vi "Main.vi"() -> ()   [LabVIEW 2013]
uses:
  <vilib>/Analysis/NI_AALBase.lvlib
  <vilib>/Analysis/1siggen.llb/Ramp Pattern by Samples.vi
  <vilib>/DAQmx/create/channels.llb/DAQmx Create Channel (AO-Voltage-Basic).vi
  <vilib>/DAQmx/write.llb/DAQmx Write (Analog 1D DBL NChan 1Samp).vi
panel:
  in  "Define as center":bool
  out "Voltage out":dbl[](array[numeric])
  in  "Relative Position":cluster{"X":i32, "Y":i32, "Z":i32}
  in  "Voltage Step":cluster{"X":dbl, "Y":dbl, "Z":dbl}
  in  "Center Voltage":cluster{"X":dbl, "Y":dbl, "Z":dbl}
  in  "2nd Dim":u32
  in  "3rd Dim":u32
  out "Intensity Graph":dbl[][](graph)
  out "XY Graph":T1(graph)
  out "Scanning":bool
  out "Estimated Time (ms)":dbl
  in  "dt (in tc)":u32
  in  "Dim3Scan":cluster{"Start":dbl, "Stop":dbl, "Steps":u32}
  in  "Dim3":u16(ring) items=["Z", "none"]
  in  "Dim2Scan":cluster{"Start":dbl, "Stop":dbl, "Steps":u32}
  in  "Dim2":u16(ring) items=["Y", "Z", "none"]
  in  "Dim1Scan":cluster{"Start":dbl, "Stop":dbl, "Steps":u32}
  in  "Dim1":u16(ring) items=["X", "Y", "Z"]
  in  "Start Scan":bool
  out "Error":errorcluster
  out "History Graph":cluster{dbl[], dbl[]}(graph)
  in  "N":u32
  out "Value":dbl
  in  "tc (ms)":u32
  in  "stop":bool
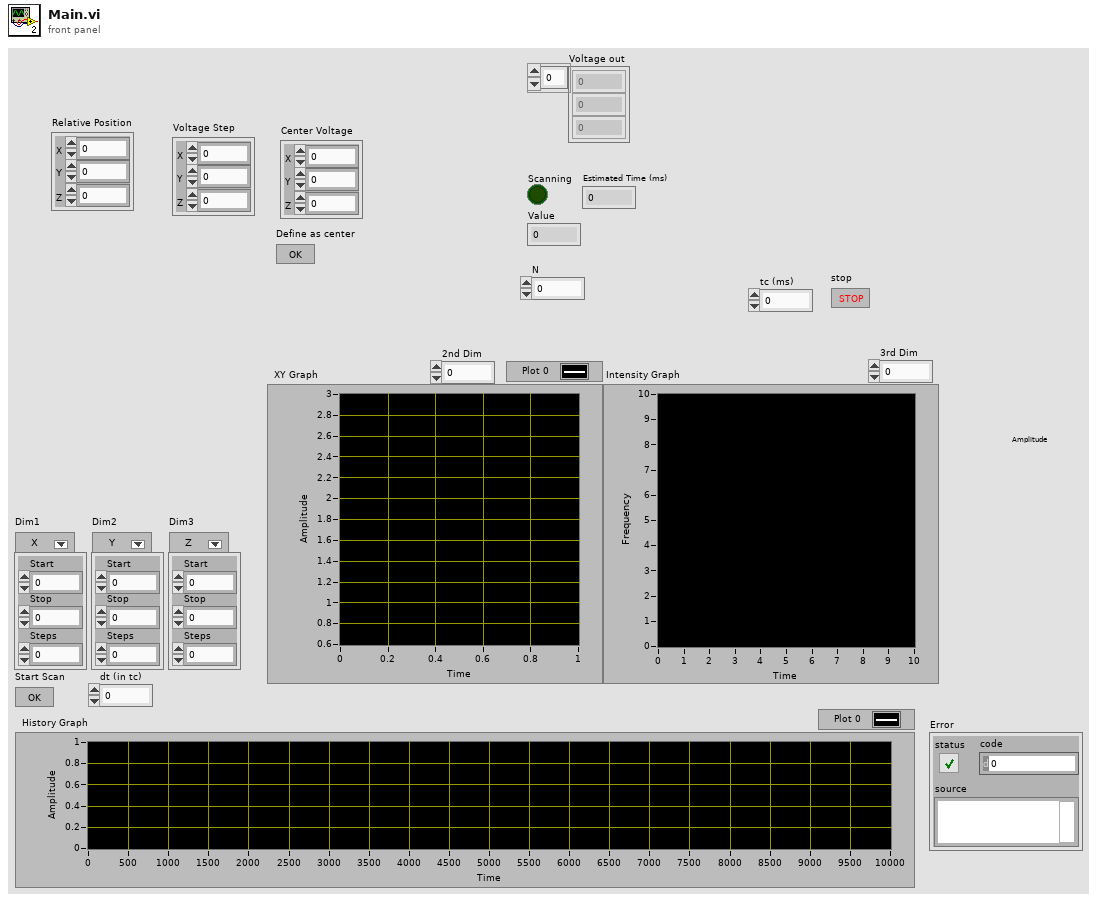
[diagram p1: front panel]
types:
  T1 = cluster{"Ramp Pattern":dbl[], "Ramp Pattern":dbl[]}
  T2 = enum16{"open", "replace", "create", "open or create", "replace or create", "replace or create with confirmation"}
  T3 = cluster{"Ramp Pattern":dbl[], "initialized array":dbl[]}
  T4 = cluster{"Voltage out[0]":dbl, "Voltage out[1]":dbl, "Voltage out[2]":dbl}
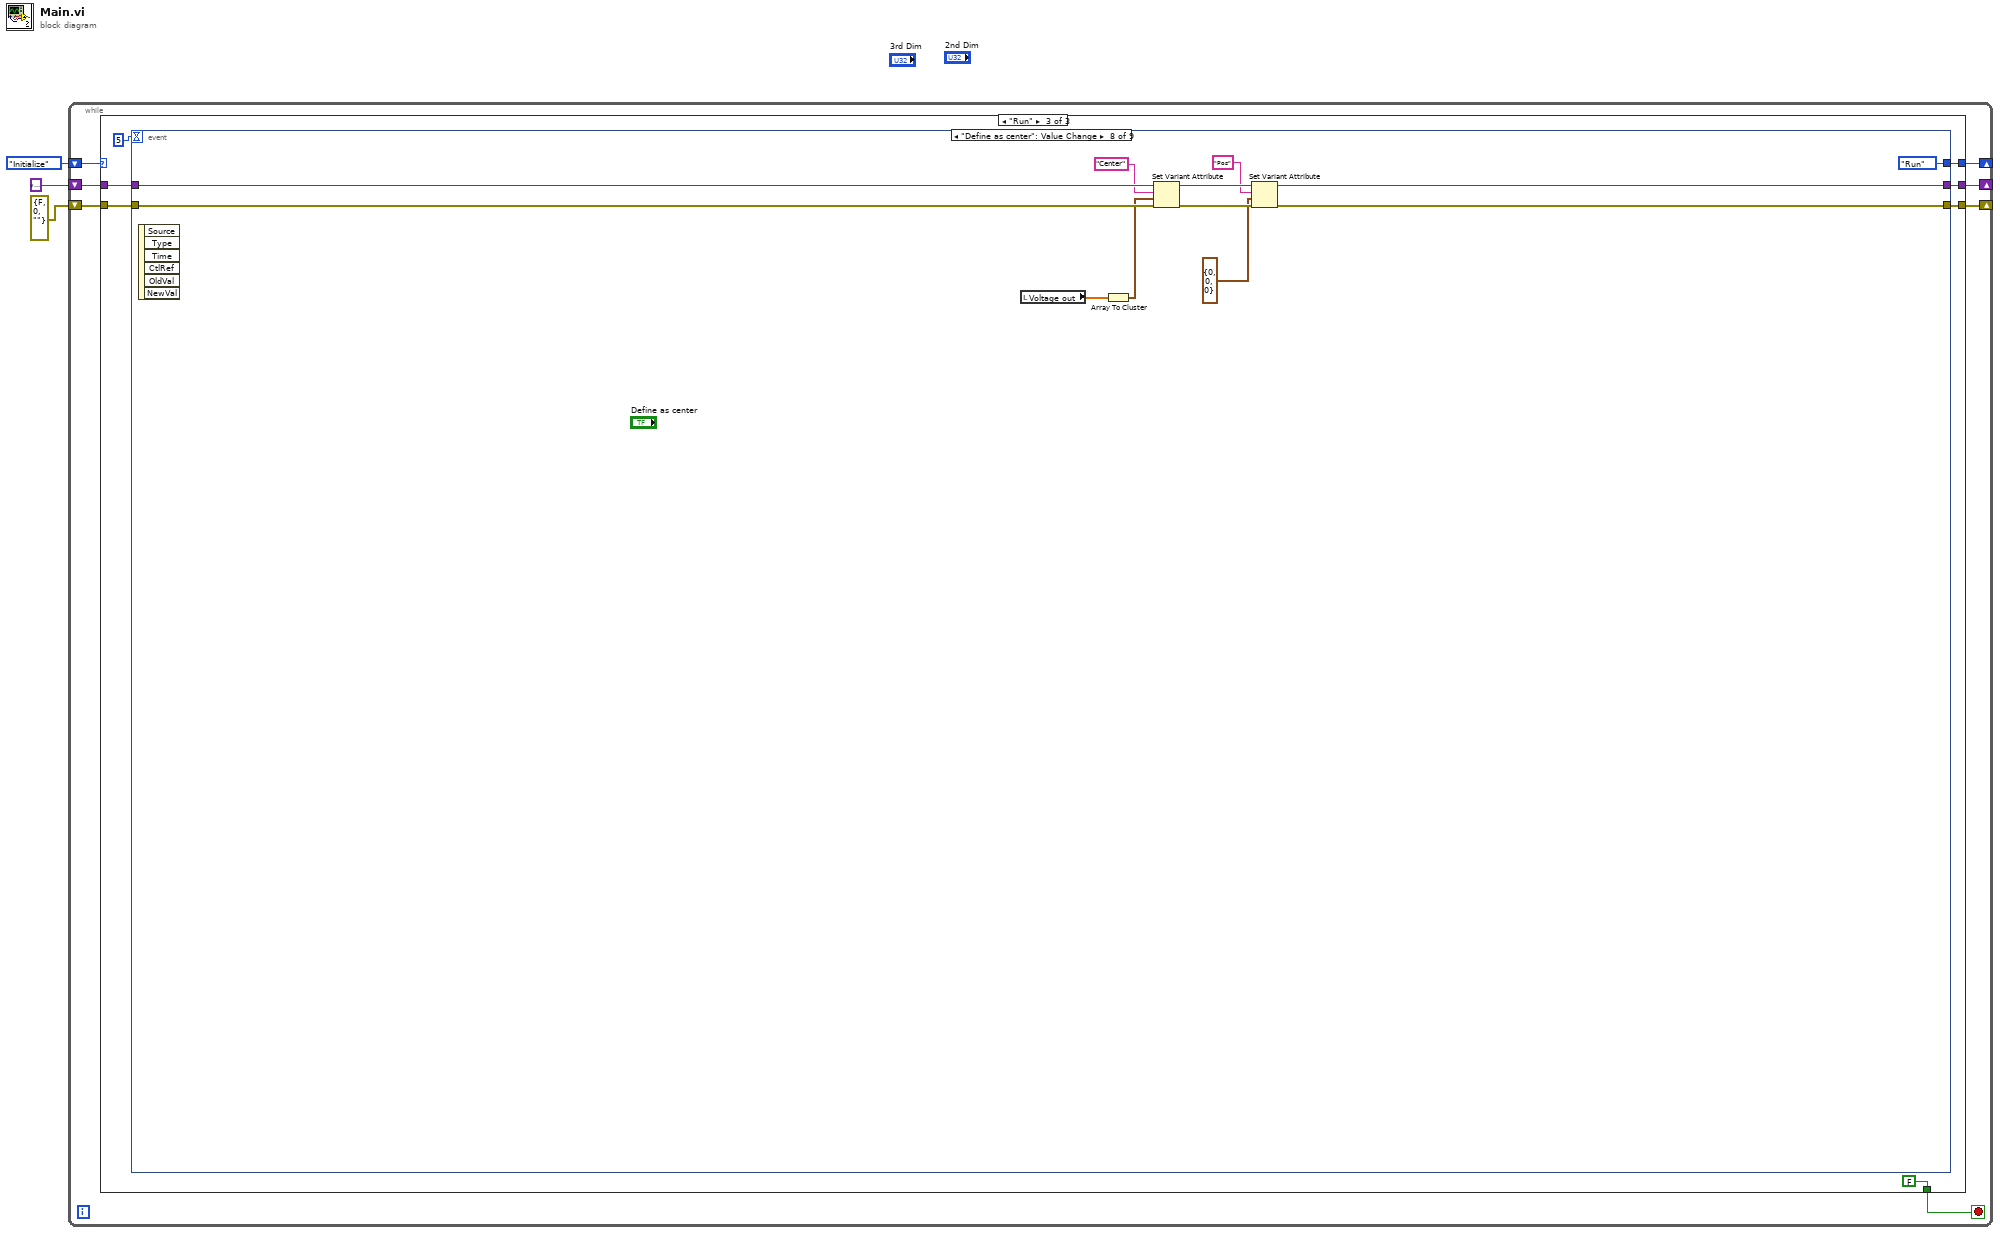
[diagram p0: block diagram]
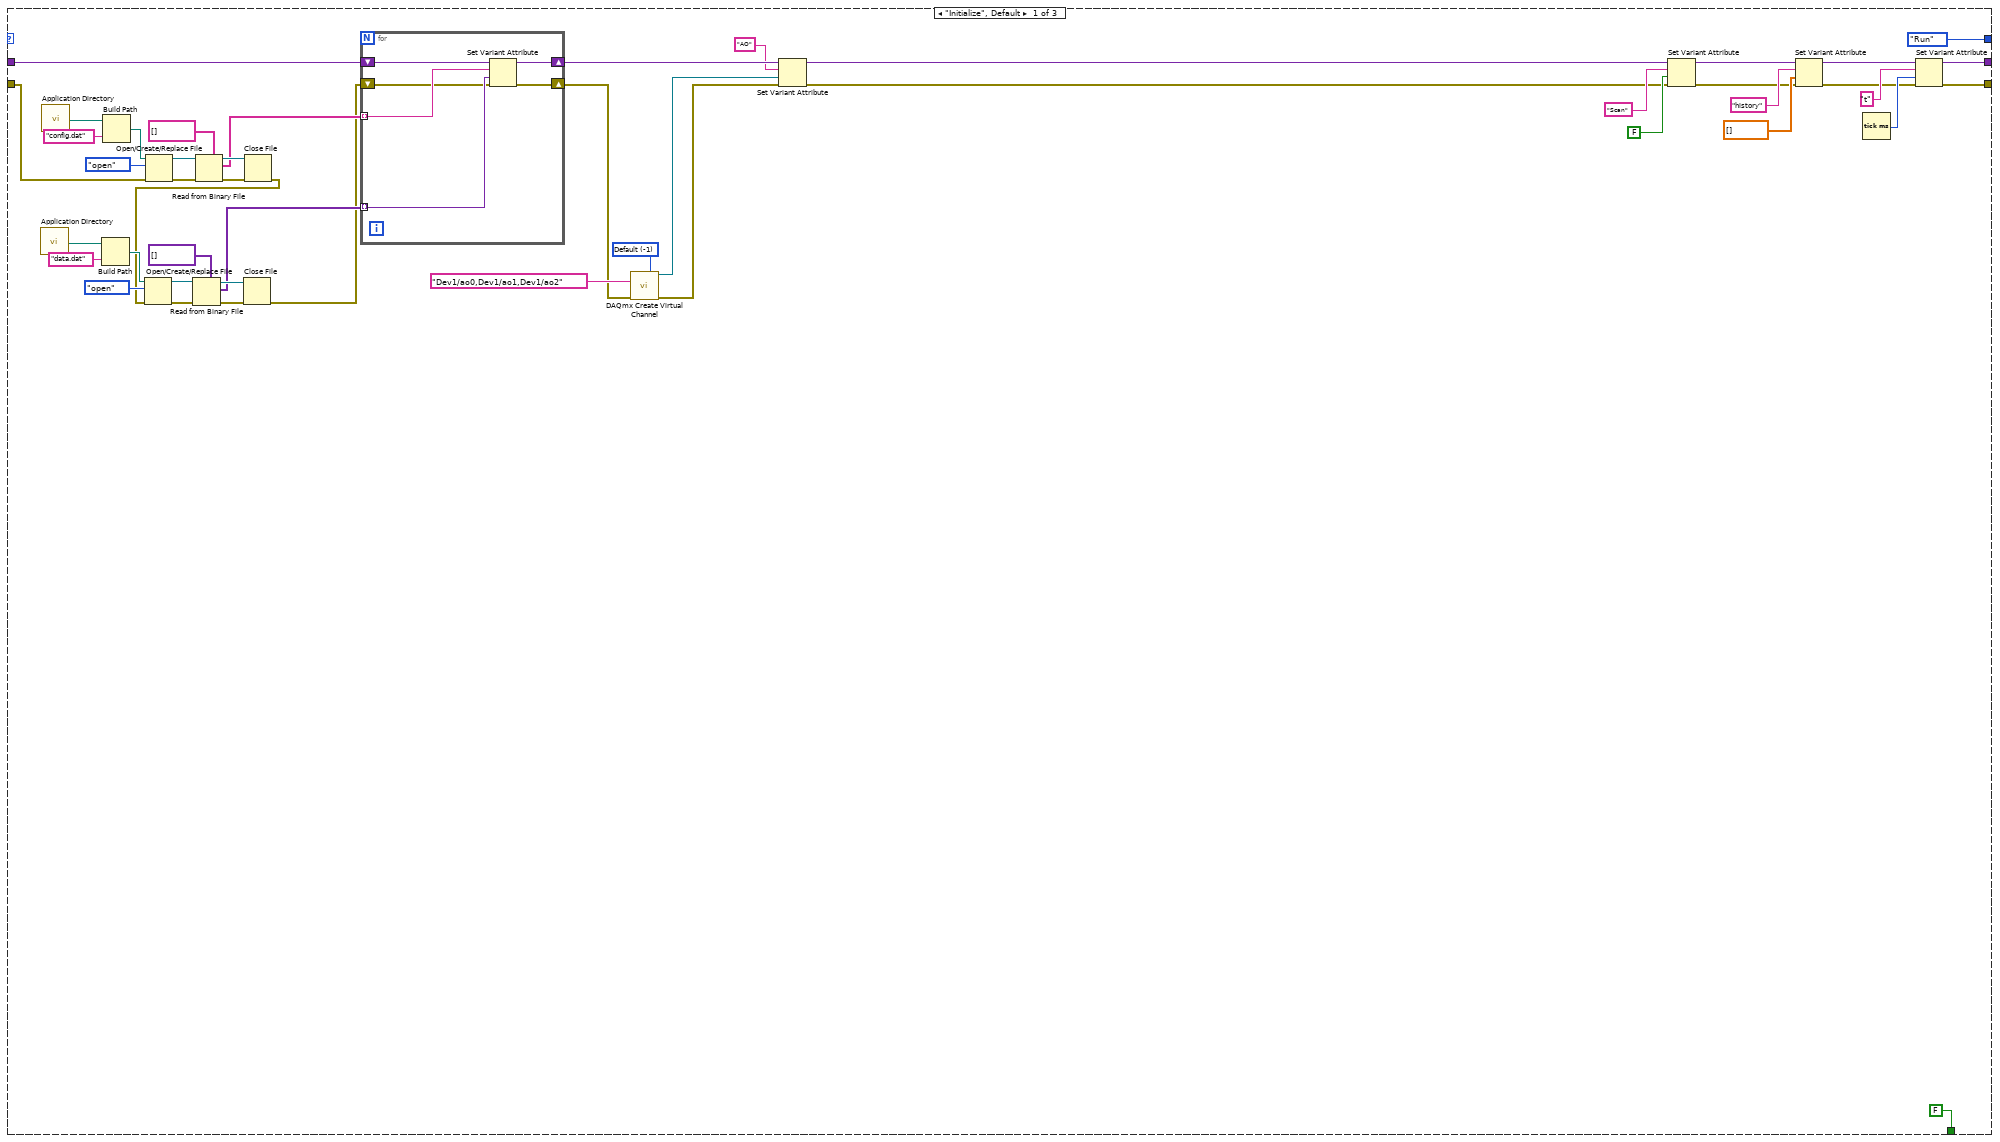
[diagram p2: hidden frame]
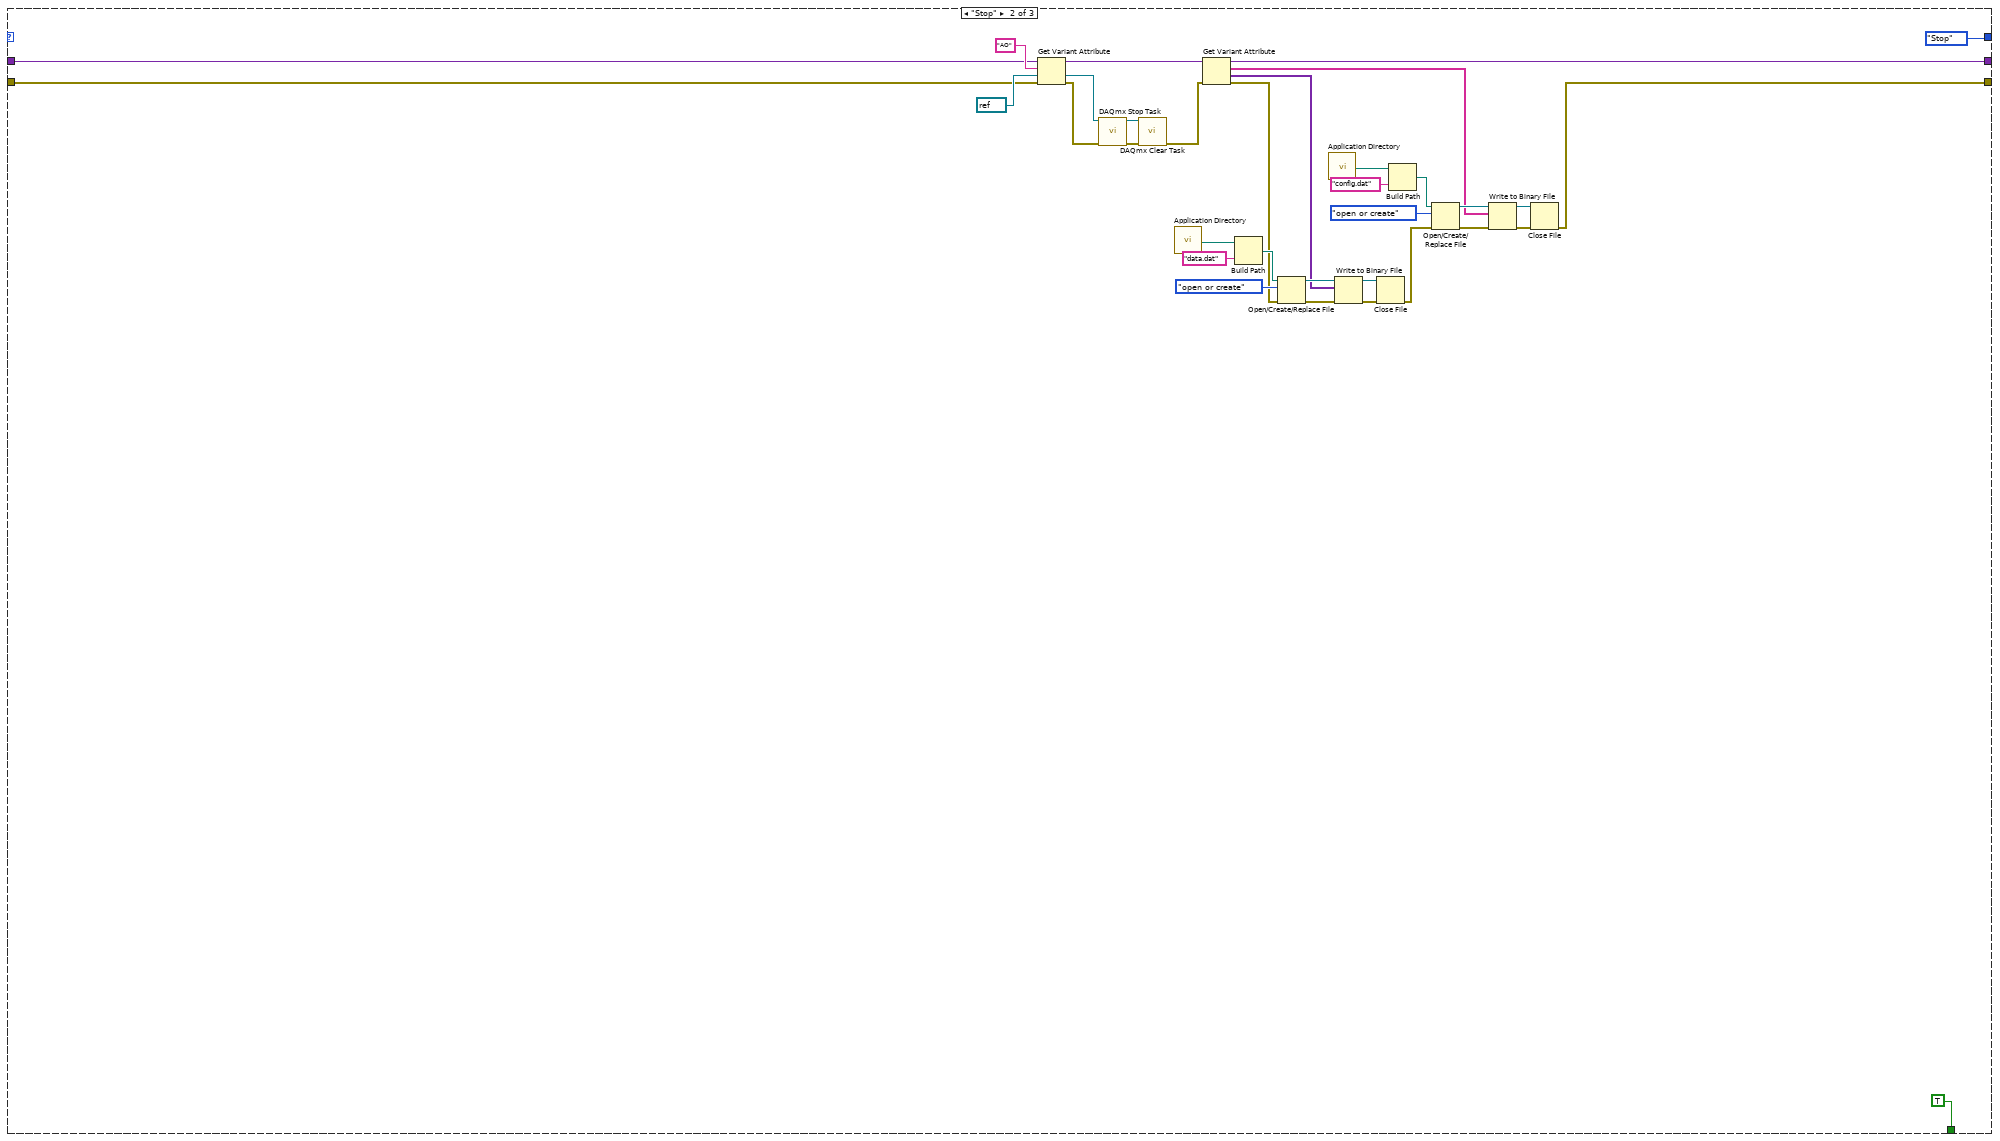
[diagram p3: hidden frame]
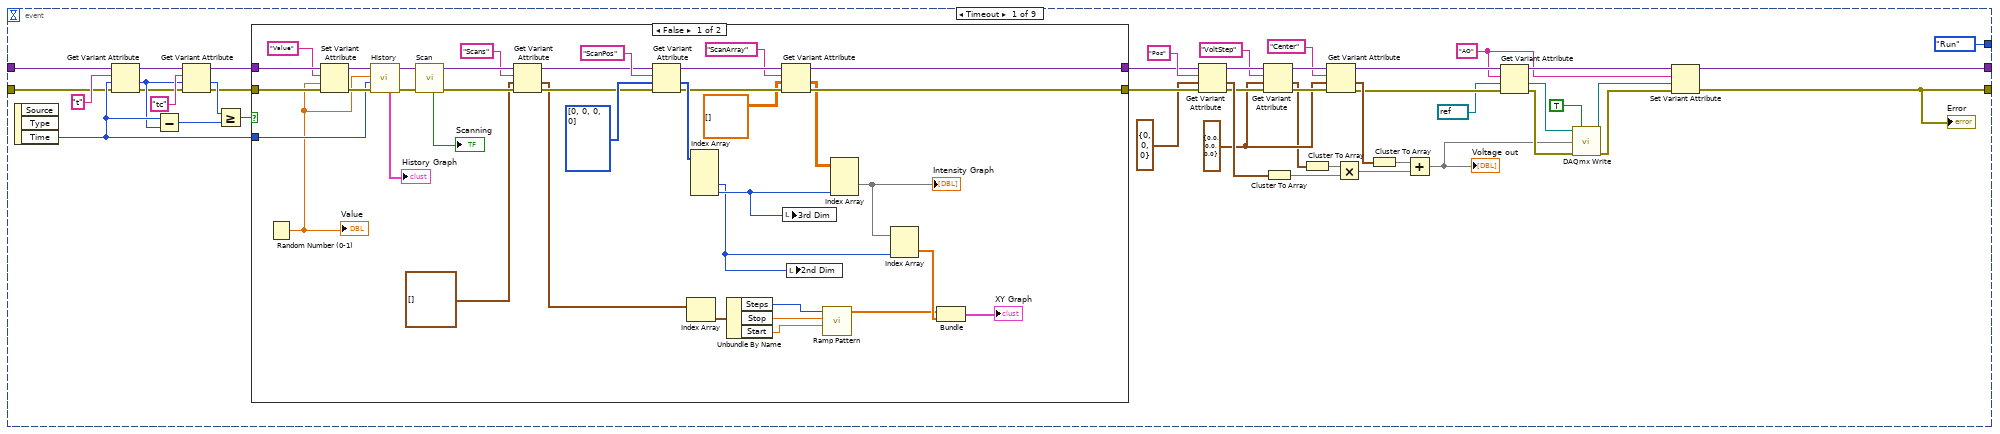
[diagram p4: hidden frame]
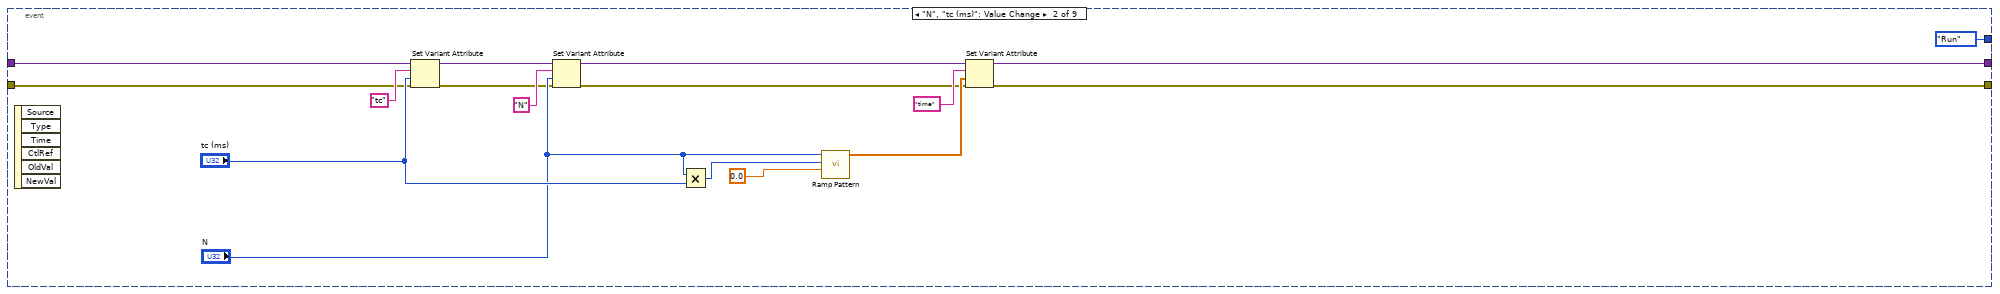
[diagram p6: hidden frame]
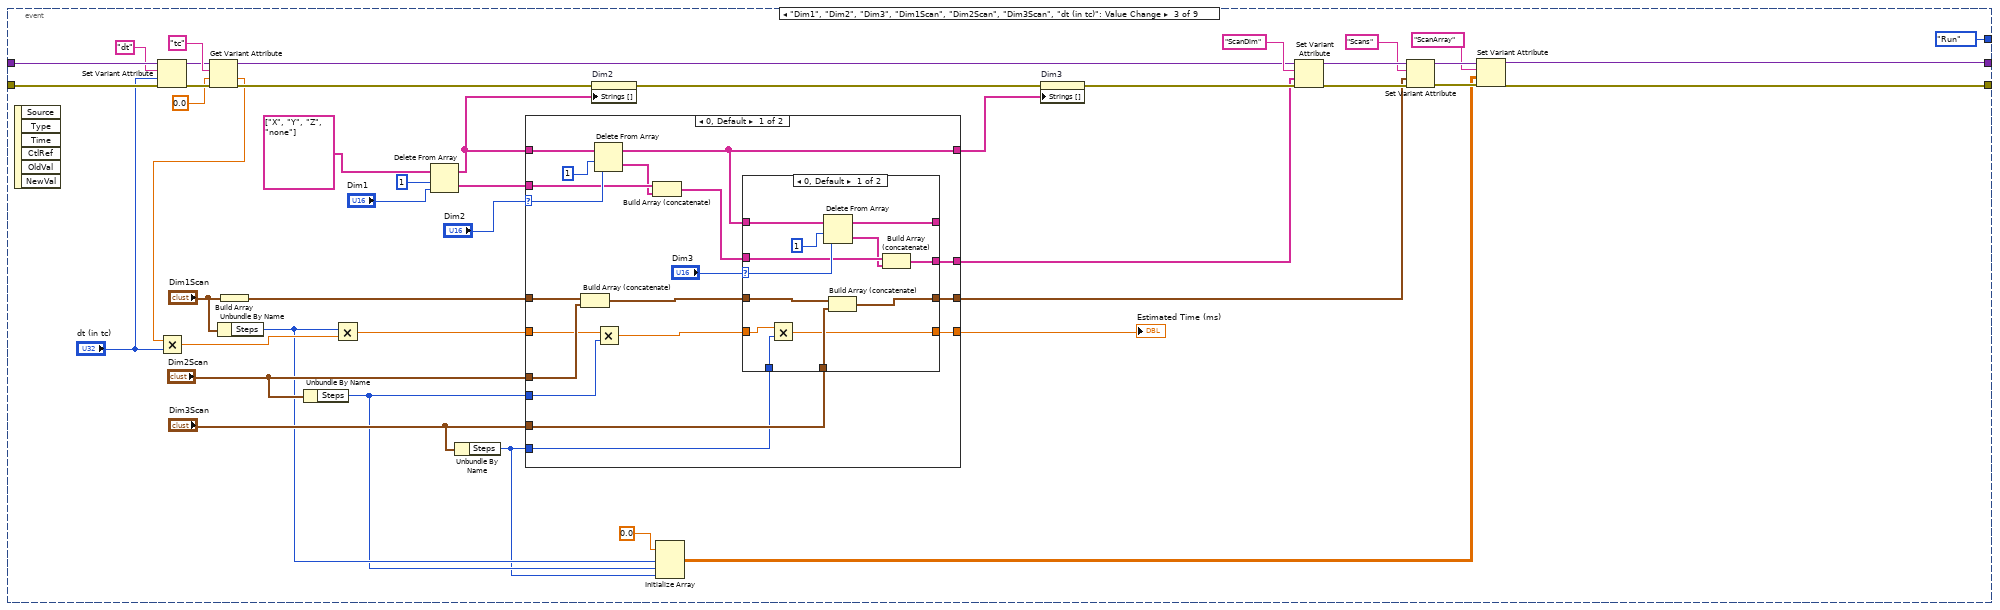
[diagram p7: hidden frame]
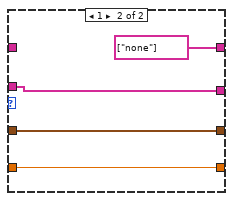
[diagram p8: hidden frame]
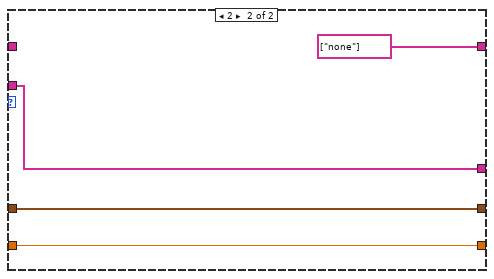
[diagram p9: hidden frame]
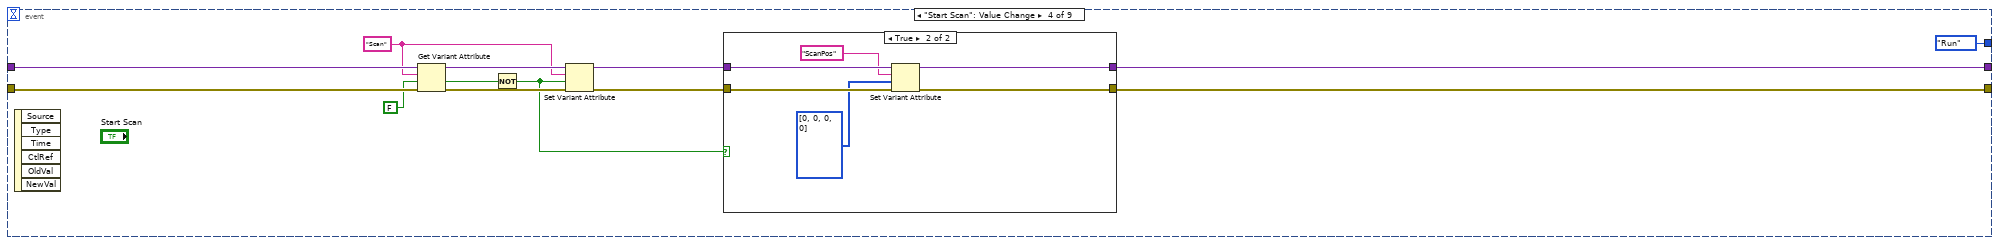
[diagram p10: hidden frame]
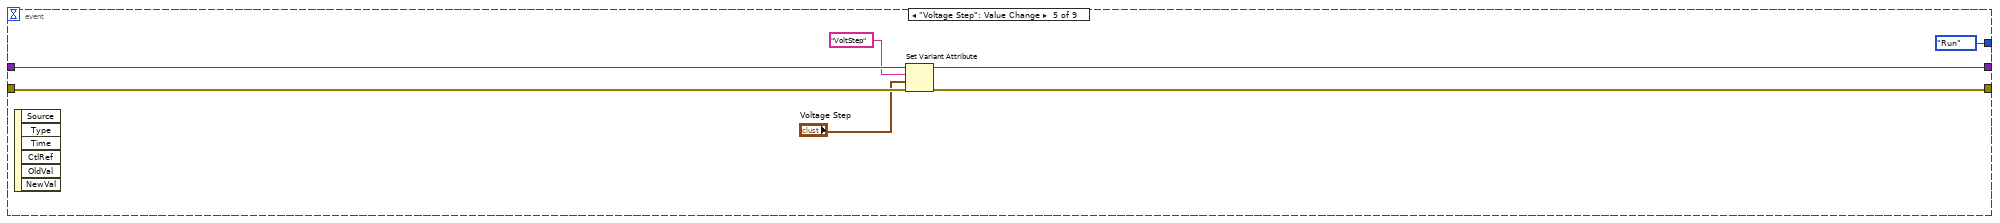
[diagram p12: hidden frame]
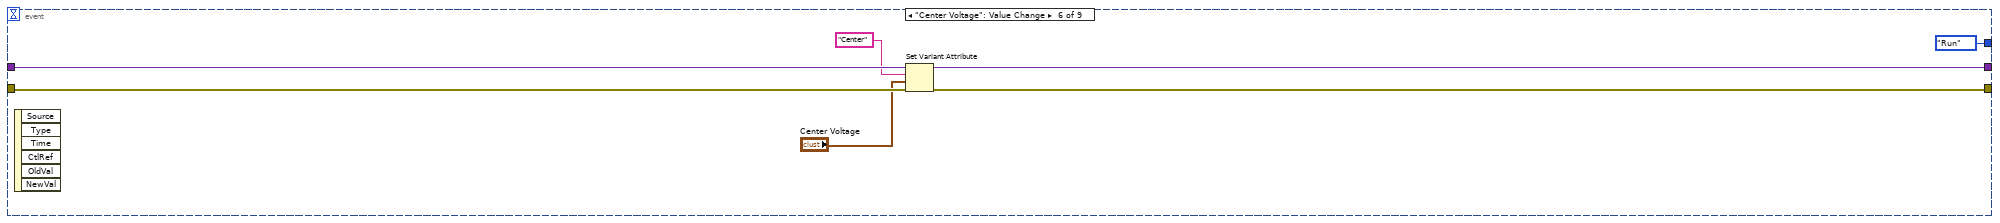
[diagram p13: hidden frame]
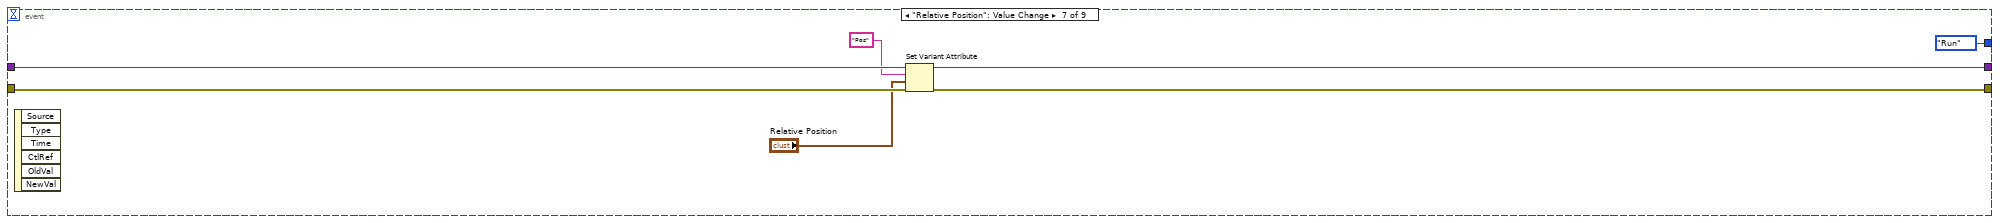
[diagram p14: hidden frame]
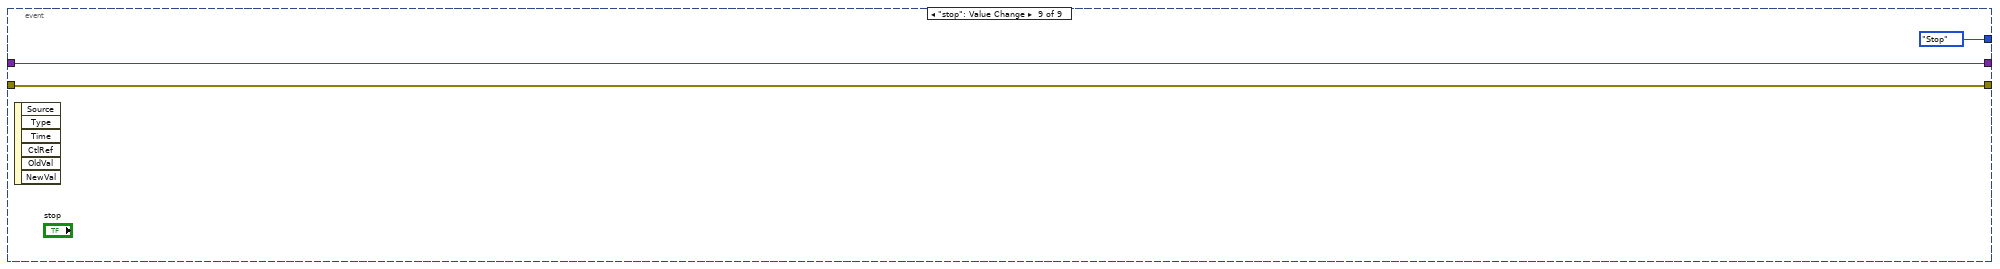
[diagram p15: hidden frame]
diagram:
  n1 = while {
    shift-right: [w9] -> _
    shift-left: enum16{"Initialize", "Run", "Stop"}."Initialize" -> [w10]
    shift-right: [w5] -> _
    shift-left: variant ("variant") -> [w7]
    shift-right: [w4] -> _
    shift-left: errorcluster {"status"=FALSE, "code"=0, "source"=""} ("error constant") -> [w6]
    stop <- w8 stop-if-true
    n2 = case shown="\"Run\"" w10 {
      tunnel: [enum16{"Initialize", "Run", "Stop"}."Run" enum16{"Initialize", "Run", "Stop"}."Stop" w104] -> w9
      tunnel: [FALSE TRUE FALSE] -> w8
      tunnel: w7 -> [w25 w70 w101]
      tunnel: w6 -> [w24 w69 w100]
      tunnel: [w27 w74 w99] -> w5
      tunnel: [w26 w75 w98] -> w4
      frame "Initialize", Default {
        w11 = -1 items=["Default"=-1, "RSE"=10083, "Differential"=10106, "Pseudodifferential"=12529] ("output terminal configuration")
        n3 = call <vilib>:"Application Directory.vi"() -> ("Application Directory"=w43:path)
        n4 = call <vilib>:"Application Directory.vi"() -> ("Application Directory"=w50:path)
        n5 = Build Path(base path=w43, name or relative path="data.dat") -> (appended path=w45:path)
        n6 = Build Path(base path=w50, name or relative path="config.dat") -> (appended path=w48:path)
        n7 = Open/Create/Replace File(file path (use dialog)=w48, error in=w24, operation (0:open)=T2."open") -> (refnum out=w40:refnum<file>, error out=w39:errorcluster)  [unwired: 3 in, 1 out]
        n8 = Read from Binary File(5:string[] [] ("names"), 8:w39, 11:w40) -> (0:w42:errorcluster, 2:w32:string[], 3:w41:refnum<file>)  [unwired: 3 in, 1 out]
        n9 = Close File(refnum=w41, error in=w42) -> (error out=w29:errorcluster)  [unwired: 1 out]
        n10 = Open/Create/Replace File(file path (use dialog)=w45, error in=w29, operation (0:open)=T2."open") -> (refnum out=w37:refnum<file>, error out=w38:errorcluster)  [unwired: 3 in, 1 out]
        n11 = Read from Binary File(5:variant[] [] ("values"), 8:w38, 11:w37) -> (0:w35:errorcluster, 2:w31:variant[], 3:w36:refnum<file>)  [unwired: 3 in, 1 out]
        n12 = Close File(refnum=w36, error in=w35) -> (error out=w28:errorcluster)  [unwired: 1 out]
        n13 = for {
          tunnel: w32 -> [w61] mode=indexing
          tunnel: w31 -> [w60] mode=indexing
          shift-right: [w62] -> w17
          shift-left: w25 -> [w63]
          shift-right: [w59] -> w18
          shift-left: w28 -> [w58]
          n14 = Set Variant Attribute(Variant=w63, name=w61, value=w60, error in=w58) -> (Variant out=w62:variant, error out=w59:errorcluster)  [unwired: 1 out]
        }
        n15 = call-poly <vilib>:"DAQmx Create Virtual Channel.vi"("output terminal configuration"=w11, "physical channels"=tag "Dev1/ao0,Dev1/ao1,Dev1/ao2", "error in"=w18) -> ("task out"=w15:refnum<k21>, "error out"=w16:errorcluster)  [unwired: 11 in]
        n16 = Set Variant Attribute(Variant=w17, name="AO", value=w15, error in=w16) -> (Variant out=w13:variant, error out=w12:errorcluster)  [unwired: 1 out]
        n17 = Set Variant Attribute(Variant=w13, name="Scan", value=FALSE, error in=w12) -> (Variant out=w23:variant, error out=w22:errorcluster)  [unwired: 1 out]
        n18 = Set Variant Attribute(Variant=w23, name="history", value=dbl[] [], error in=w22) -> (Variant out=w53:variant, error out=w30:errorcluster)  [unwired: 1 out]
        n19 = Tick Count (ms)() -> (millisecond timer value=w54:u32)
        n20 = Set Variant Attribute(Variant=w53, name="t", value=w54, error in=w30) -> (Variant out=w27:variant, error out=w26:errorcluster)  [unwired: 1 out]
      }
      frame "Stop" {
        n21 = Get Variant Attribute(Variant=w70, name="AO", default value (empty Variant)=refnum<k21> refnum ("task out"), error in=w69) -> (duplicate Variant=w71:variant, value=w64:refnum<k21>, error out=w66:errorcluster)  [unwired: 1 out]
        n22 = call <vilib>:"DAQmx Stop Task.vi"("task/channels in"=w64, "error in"=w66) -> ("task out"=w68:refnum<k21>, "error out"=w67:errorcluster)  [unwired: 12 in]
        n23 = call <vilib>:"DAQmx Clear Task.vi"("task in"=w68, "error in"=w67) -> ("error out"=w65:errorcluster)  [unwired: 13 in]
        n24 = call <vilib>:"Application Directory.vi"() -> ("Application Directory"=w88:path)
        n25 = Get Variant Attribute(Variant=w71, error in=w65) -> (duplicate Variant=w74:variant, names=w78:string[], values=w87:variant[], error out=w77:errorcluster)  [unwired: 2 in]
        n26 = Build Path(base path=w88, name or relative path="data.dat") -> (appended path=w94:path)
        n27 = Open/Create/Replace File(file path (use dialog)=w94, error in=w77, operation (0:open)=T2."open or create") -> (refnum out=w93:refnum<file>, error out=w90:errorcluster)  [unwired: 3 in, 1 out]
        n28 = call <vilib>:"Application Directory.vi"() -> ("Application Directory"=w86:path)
        n29 = Write to Binary File(file (use dialog)=w93, data=w87, error in=w90) -> (refnum out=w91:refnum<file>, error out=w89:errorcluster)  [unwired: 3 in, 1 out]
        n30 = Close File(refnum=w91, error in=w89) -> (error out=w76:errorcluster)  [unwired: 1 out]
        n31 = Build Path(base path=w86, name or relative path="config.dat") -> (appended path=w80:path)
        n32 = Open/Create/Replace File(file path (use dialog)=w80, error in=w76, operation (0:open)=T2."open or create") -> (refnum out=w81:refnum<file>, error out=w84:errorcluster)  [unwired: 3 in, 1 out]
        n33 = Write to Binary File(file (use dialog)=w81, data=w78, error in=w84) -> (refnum out=w83:refnum<file>, error out=w85:errorcluster)  [unwired: 3 in, 1 out]
        n34 = Close File(refnum=w83, error in=w85) -> (error out=w75:errorcluster)  [unwired: 1 out]
      }
      frame "Run" {
        n35 = event shown="[7] \"Define as center\": Value Change" {
          selector: _ -> [_ _ _ _ _ _ _ _ _]
          dyn-events: _ -> [_ _ _ _ _ _ _ _ _]
          timeout: 5 -> [_ _ _ _ _ _ _ _ _]
          tunnel: [enum16{"Initialize", "Run", "Stop"}."Run" enum16{"Initialize", "Run", "Stop"}."Run" enum16{"Initialize", "Run", "Stop"}."Run" enum16{"Initialize", "Run", "Stop"}."Run" enum16{"Initialize", "Run", "Stop"}."Run" enum16{"Initialize", "Run", "Stop"}."Run" enum16{"Initialize", "Run", "Stop"}."Run" enum16{"Initialize", "Run", "Stop"}."Run" enum16{"Initialize", "Run", "Stop"}."Stop"] -> w104
          tunnel: w101 -> [w139 w193 w235 w302 w317 w324 w331 w343 w346]
          tunnel: w100 -> [w138 w192 w234 w301 w316 w323 w330 w341 w345]
          tunnel: [w106 w191 w210 w292 w315 w322 w329 w340 w346] -> w99
          tunnel: [w105 w190 w209 w291 w314 w321 w328 w339 w345] -> w98
          event Timeout {
            w107 = "AO" ("name")
            w124 = cluster{"X":dbl, "Y":dbl, "Z":dbl} {"X"=0.0, "Y"=0.0, "Z"=0.0} ("Relative Position")
            n36 = event-data() -> ("Time"=w145:u32)  [unwired: 1 in, 2 out]
            n37 = Get Variant Attribute(Variant=w139, name="t", default value (empty Variant)=w145, error in=w138) -> (duplicate Variant=w144:variant, value=w142:u32, error out=w140:errorcluster)  [unwired: 1 out]
            n38 = Subtract(x=w145, y=w142) -> (x-y=w147:u32)
            n39 = Get Variant Attribute(Variant=w144, name="tc", default value (empty Variant)=w142, error in=w140) -> (duplicate Variant=w137:variant, value=w141:u32, error out=w136:errorcluster)  [unwired: 1 out]
            n40 = Greater Or Equal?(x=w141, y=w147) -> (x >= y?=w146:bool)
            n41 = case shown="False" w146 {
              tunnel: w145 -> [w181 _]
              tunnel: w137 -> [w187 w189]
              tunnel: w136 -> [w186 w188]
              tunnel: [w171 w189] -> w134
              tunnel: [w170 w188] -> w133
              frame False {
                n42 = Random Number (0-1)() -> (number: 0 to 1=w180:dbl)
                "Value" <- w180
                n43 = Set Variant Attribute(Variant=w187, name="Value", value=w180, error in=w186) -> (Variant out=w183:variant, error out=w184:errorcluster)  [unwired: 1 out]
                n44 = call "History.vi"("error in"=w184, "time"=w181, "Value"=w180, "variant in"=w183) -> ("error out"=w178:errorcluster, "variant out"=w179:variant, "history graph"=→"History Graph":cluster{dbl[], dbl[]})  [unwired: 5 in]
                n45 = call "Scan.vi"("error in"=w178, "variant in"=w179) -> ("error out"=w164:errorcluster, "variant out"=w165:variant, "Scanning"=→"Scanning":bool)  [unwired: 7 in]
                n46 = Get Variant Attribute(Variant=w165, name="Scans", default value (empty Variant)=cluster{"Start":dbl, "Stop":dbl, "Steps":u32}[] [], error in=w164) -> (duplicate Variant=w163:variant, value=w159:cluster{"Start":dbl, "Stop":dbl, "Steps":u32}[], error out=w162:errorcluster)  [unwired: 1 out]
                n47 = Get Variant Attribute(Variant=w163, name="ScanPos", default value (empty Variant)=i32[] [0, 0, 0, 0], error in=w162) -> (duplicate Variant=w173:variant, value=w174:i32[], error out=w172:errorcluster)  [unwired: 1 out]
                n48 = Index Array(array=w159) -> (element=w158:cluster{"Start":dbl, "Stop":dbl, "Steps":u32})  [unwired: 1 in]
                n49 = Index Array(array=w174) -> (element #3=w150:i32, element #4=w151:i32)  [unwired: 4 in, 2 out]
                n50 = Unbundle By Name(w158) -> ("Steps"=w157:u32, "Stop"=w156:dbl, "Start"=w155:dbl)
                n51 = Get Variant Attribute(Variant=w173, name="ScanArray", default value (empty Variant)=dbl[][][] [] ("initialized array"), error in=w172) -> (duplicate Variant=w171:variant, value=w167:dbl[][][], error out=w170:errorcluster)  [unwired: 1 out]
                n52 = local write "3rd Dim"(w151) -> ()
                n53 = local write "2nd Dim"(w150) -> ()
                n54 = call-poly <vilib>:"Ramp Pattern.vi"("start"=w155, "end"=w156, "samples"=w157) -> ("Ramp Pattern"=w152:dbl[])  [unwired: 7 in, 1 out]
                n55 = Index Array(array=w167, index (dim 2)=w151) -> (element=w166:dbl[][])  [unwired: 2 in]
                "Intensity Graph" <- w166
                n56 = Index Array(array=w166, index (col)=w150) -> (element=w153:dbl[])  [unwired: 1 in]
                n57 = Bundle("Ramp Pattern"=w152, "initialized array"=w153) -> (→"XY Graph":T3)  [unwired: 1 in]
              }
              frame True {
              }
            }
            n58 = Get Variant Attribute(Variant=w134, name="Pos", default value (empty Variant)=cluster{"X":i32, "Y":i32, "Z":i32} {"X"=0, "Y"=0, "Z"=0} ("Relative Position"), error in=w133) -> (duplicate Variant=w130:variant, value=w131:cluster{"X":i32, "Y":i32, "Z":i32}, error out=w129:errorcluster)  [unwired: 1 out]
            n59 = Get Variant Attribute(Variant=w130, name="VoltStep", default value (empty Variant)=w124, error in=w129) -> (duplicate Variant=w128:variant, value=w123:cluster{"X":dbl, "Y":dbl, "Z":dbl}, error out=w127:errorcluster)  [unwired: 1 out]
            n60 = Cluster To Array(cluster=w131) -> (array=w120:i32[])
            n61 = Cluster To Array(cluster=w123) -> (array=w121:dbl[])
            n62 = Get Variant Attribute(Variant=w128, name="Center", default value (empty Variant)=w124, error in=w127) -> (duplicate Variant=w117:variant, value=w122:cluster{"X":dbl, "Y":dbl, "Z":dbl}, error out=w116:errorcluster)  [unwired: 1 out]
            n63 = Multiply(x=w121, y=w120) -> (x*y=w118:dbl[])
            n64 = Cluster To Array(cluster=w122) -> (array=w119:dbl[])
            n65 = Add(x=w119, y=w118) -> (x+y=w112:dbl[])
            "Voltage out" <- w112
            n66 = Get Variant Attribute(Variant=w117, name=w107, default value (empty Variant)=refnum<k21> refnum ("task out"), error in=w116) -> (duplicate Variant=w109:variant, value=w114:refnum<k21>, error out=w113:errorcluster)  [unwired: 1 out]
            n67 = call-poly <vilib>:"DAQmx Write.vi"("task/channels in"=w114, "auto start"=TRUE, "data"=w112, "error in"=w113) -> ("task out"=w108:refnum<k21>, "error out"=w110:errorcluster)  [unwired: 9 in, 1 out]
            n68 = Set Variant Attribute(Variant=w109, name=w107, value=w108, error in=w110) -> (Variant out=w106:variant, error out=w105:errorcluster)  [unwired: 1 out]
            "Error" <- w105
          }
          event "N", "tc (ms)": Value Change {
            n69 = event-data() -> ()  [unwired: 1 in, 6 out]
            n70 = Set Variant Attribute(Variant=w193, name="tc", value="tc (ms)", error in=w192) -> (Variant out=w206:variant, error out=w195:errorcluster)  [unwired: 1 out]
            n71 = Set Variant Attribute(Variant=w206, name="N", value="N", error in=w195) -> (Variant out=w199:variant, error out=w194:errorcluster)  [unwired: 1 out]
            n72 = Multiply(x="N", y="tc (ms)") -> (x*y=w201:u32)
            n73 = call-poly <vilib>:"Ramp Pattern.vi"("start"=0.0, "end"=w201, "samples"="N") -> ("Ramp Pattern"=w197:dbl[])  [unwired: 7 in, 1 out]
            n74 = Set Variant Attribute(Variant=w199, name="time", value=w197, error in=w194) -> (Variant out=w191:variant, error out=w190:errorcluster)  [unwired: 1 out]
          }
          event "Dim1", "Dim2", "Dim3", "Dim1Scan", "Dim2Scan", "Dim3Scan", "dt (in tc)": Value Change {
            n75 = event-data() -> ()  [unwired: 1 in, 6 out]
            n76 = Set Variant Attribute(Variant=w235, name="dt", value="dt (in tc)", error in=w234) -> (Variant out=w224:variant, error out=w223:errorcluster)  [unwired: 1 out]
            n77 = Get Variant Attribute(Variant=w224, name="tc", default value (empty Variant)=0.0, error in=w223) -> (duplicate Variant=w221:variant, value=w220:dbl, error out=w222:errorcluster)  [unwired: 1 out]
            n78 = Multiply(x=w220, y="dt (in tc)") -> (x*y=w218:dbl)
            n79 = Unbundle By Name("Dim1Scan") -> ("Steps"=w215:u32)
            n80 = Build Array("Dim1Scan") -> (w241:cluster{"Start":dbl, "Stop":dbl, "Steps":u32}[])
            n81 = Unbundle By Name("Dim2Scan") -> ("Steps"=w214:u32)
            n82 = Multiply(x=w215, y=w218) -> (x*y=w237:dbl)
            n83 = Delete From Array(array=string[] ["X", "Y", "Z", "none"], length=1, index="Dim1") -> (deleted portion=w243:string[], array with subset deleted=w244:string[])
            n84 = Unbundle By Name("Dim3Scan") -> ("Steps"=w213:u32)
            n85 = case shown="0, Default" "Dim2" {
              selector: "Dim2" -> [w268 _]
              tunnel: [w262 string[] ["none"] ("Strings []")] -> w242
              tunnel: w244 -> [w267 _]
              tunnel: w243 -> [w266 w289]
              tunnel: [w261 w289] -> w227
              tunnel: w241 -> [w260 w288]
              tunnel: [w256 w288] -> w226
              tunnel: "Dim2Scan" -> [w259 _]
              tunnel: "Dim3Scan" -> [w257 _]
              tunnel: w237 -> [w255 w287]
              tunnel: [w251 w287] -> w236
              tunnel: w214 -> [w254 _]
              tunnel: w213 -> [w252 _]
              frame 0, Default {
                n86 = Build Array (concatenate)(w260, w259) -> (w258:cluster{"Start":dbl, "Stop":dbl, "Steps":u32}[])
                n87 = Delete From Array(array=w267, length=1, index=w268) -> (deleted portion=w265:string[], array with subset deleted=w262:string[])
                n88 = Multiply(x=w255, y=w254) -> (x*y=w253:dbl)
                n89 = Build Array (concatenate)(w266, w265) -> (w263:string[])
                n90 = case shown="0, Default" "Dim3" {
                  selector: "Dim3" -> [w281 _]
                  tunnel: [w277 string[] ["none"] ("Strings []")] -> _
                  tunnel: w263 -> [w280 w285]
                  tunnel: [w279 w285] -> w261
                  tunnel: w262 -> [w278 _]
                  tunnel: w258 -> [w275 w284]
                  tunnel: w257 -> [w274 _]
                  tunnel: [w273 w284] -> w256
                  tunnel: w253 -> [w272 w283]
                  tunnel: w252 -> [w271 _]
                  tunnel: [w270 w283] -> w251
                  frame 0, Default {
                    n91 = Multiply(x=w272, y=w271) -> (x*y=w270:dbl)
                    n92 = Delete From Array(array=w278, length=1, index=w281) -> (deleted portion=w276:string[], array with subset deleted=w277:string[])
                    n93 = Build Array (concatenate)(w275, w274) -> (w273:cluster{"Start":dbl, "Stop":dbl, "Steps":u32}[])
                    n94 = Build Array (concatenate)(w280, w276) -> (w279:string[])
                  }
                  frame 1 {
                  }
                }
              }
              frame 2 {
              }
            }
            "Estimated Time (ms)" <- w236
            n95 = property on="Dim2" class="Ring (strict)"(error in=w222, "Strings []"=w244) -> (error out=w245:errorcluster)  [unwired: 1 in, 1 out]
            n96 = Initialize Array(0.0, w215, w214, w213) -> (w207:dbl[][][])
            n97 = property on="Dim3" class="Ring (strict)"(error in=w245, "Strings []"=w242) -> (error out=w231:errorcluster)  [unwired: 1 in, 1 out]
            n98 = Set Variant Attribute(Variant=w221, name="ScanDim", value=w227, error in=w231) -> (Variant out=w233:variant, error out=w232:errorcluster)  [unwired: 1 out]
            n99 = Set Variant Attribute(Variant=w233, name="Scans", value=w226, error in=w232) -> (Variant out=w212:variant, error out=w211:errorcluster)  [unwired: 1 out]
            n100 = Set Variant Attribute(Variant=w212, name="ScanArray", value=w207, error in=w211) -> (Variant out=w210:variant, error out=w209:errorcluster)  [unwired: 1 out]
          }
          event "Start Scan": Value Change {
            w298 = "Scan" ("name")
            n101 = event-data() -> ()  [unwired: 1 in, 6 out]
            n102 = Get Variant Attribute(Variant=w302, name=w298, default value (empty Variant)=FALSE, error in=w301) -> (duplicate Variant=w300:variant, value=w296:bool, error out=w299:errorcluster)  [unwired: 1 out]
            n103 = Not(x=w296) -> (.not. x?=w295:bool)
            n104 = Set Variant Attribute(Variant=w300, name=w298, value=w295, error in=w299) -> (Variant out=w294:variant, error out=w293:errorcluster)  [unwired: 1 out]
            n105 = case shown="True" w295 {
              tunnel: w294 -> [w305 w311]
              tunnel: w293 -> [w304 w310]
              tunnel: [w305 w307] -> w292
              tunnel: [w304 w306] -> w291
              frame False {
              }
              frame True {
                n106 = Set Variant Attribute(Variant=w311, name="ScanPos", value=i32[] [0, 0, 0, 0], error in=w310) -> (Variant out=w307:variant, error out=w306:errorcluster)  [unwired: 1 out]
              }
            }
          }
          event "Voltage Step": Value Change {
            n107 = event-data() -> ()  [unwired: 1 in, 6 out]
            n108 = Set Variant Attribute(Variant=w317, name="VoltStep", value="Voltage Step", error in=w316) -> (Variant out=w315:variant, error out=w314:errorcluster)  [unwired: 1 out]
          }
          event "Center Voltage": Value Change {
            n109 = event-data() -> ()  [unwired: 1 in, 6 out]
            n110 = Set Variant Attribute(Variant=w324, name="Center", value="Center Voltage", error in=w323) -> (Variant out=w322:variant, error out=w321:errorcluster)  [unwired: 1 out]
          }
          event "Relative Position": Value Change {
            n111 = event-data() -> ()  [unwired: 1 in, 6 out]
            n112 = Set Variant Attribute(Variant=w331, name="Pos", value="Relative Position", error in=w330) -> (Variant out=w329:variant, error out=w328:errorcluster)  [unwired: 1 out]
          }
          event "Define as center": Value Change {
            n113 = event-data() -> ()  [unwired: 1 in, 6 out]
            n114 = local read "Voltage out"() -> (w337:dbl[])
            n115 = Array To Cluster(array=w337) -> (cluster=w336:T4)
            n116 = Set Variant Attribute(Variant=w343, name="Center", value=w336, error in=w341) -> (Variant out=w342:variant, error out=w338:errorcluster)  [unwired: 1 out]
            n117 = Set Variant Attribute(Variant=w342, name="Pos", value=cluster{"X":i32, "Y":i32, "Z":i32} {"X"=0, "Y"=0, "Z"=0} ("Relative Position"), error in=w338) -> (Variant out=w340:variant, error out=w339:errorcluster)  [unwired: 1 out]
          }
          event "stop": Value Change {
            n118 = event-data() -> ()  [unwired: 1 in, 6 out]
          }
        }
      }
    }
  }
